vi "DHT.vi"() -> ()   [LabVIEW 2024]
uses:
  <vilib>/MakerHub/LINX/Public/Utilities/Open Serial.vi
  <vilib>/MakerHub/LINX/LMH-LINX.lvlib
panel:
  in  "FOLDER REPORTS":path
  in  "SAVE DATA":bool
  out "TOTAL ALARM OF HUM":dbl
  out "TOTAL ALARM OF TEMP":dbl
  out "REAL TIME TEMPERATURE C°":u8
  out "REAL TIME HUMIDITY %":u8
  out "ALLARME UMIDITA'":bool
  out "ALLARME TEMPERATURA":bool
  in  "INF HUMIDITY %":u16
  in  "SUP HUMIDITY %":u16
  in  "INF TEMPERATURE C°":u16
  in  "SUP TEMPERATURE C°":u16
  out "SAMPLES ACQUISITI":u16
  out "MODA T C°":dbl
  out "MINIMO T C°":dbl
  out "MODA H%":dbl
  out "MINIMO H%":dbl
  in  "SAMPLE TIME [ms]":u16=100 min=100
  out "MASSIMO T C°":dbl
  out "DEV STD T":dbl
  out "MEDIA T C°":dbl
  out "MASSIMO H%":dbl
  out "DEV STD H":dbl
  out "MEDIA H%":dbl
  out "HUMIDITY %":u8[](graph)
  out "TEMPERATURE C°":u8[](graph)
  out "COMUNICATION":string
  out "TEMPERATURE C°":u8(graph)
  out "HUMIDITY %":u8(graph)
  in  "NUMERO DI CAMPIONI":u16
  in  "ACQUIRE":bool
  in  "stop":bool
  in  "Serial Port":refnum<visa-resource-name>="N/A"
  # "SOGLIE"
  # "PARAMETRI STATISTICI TEMPERATURA"
  # "PARAMETRI STATISTICI UMIDITA'"
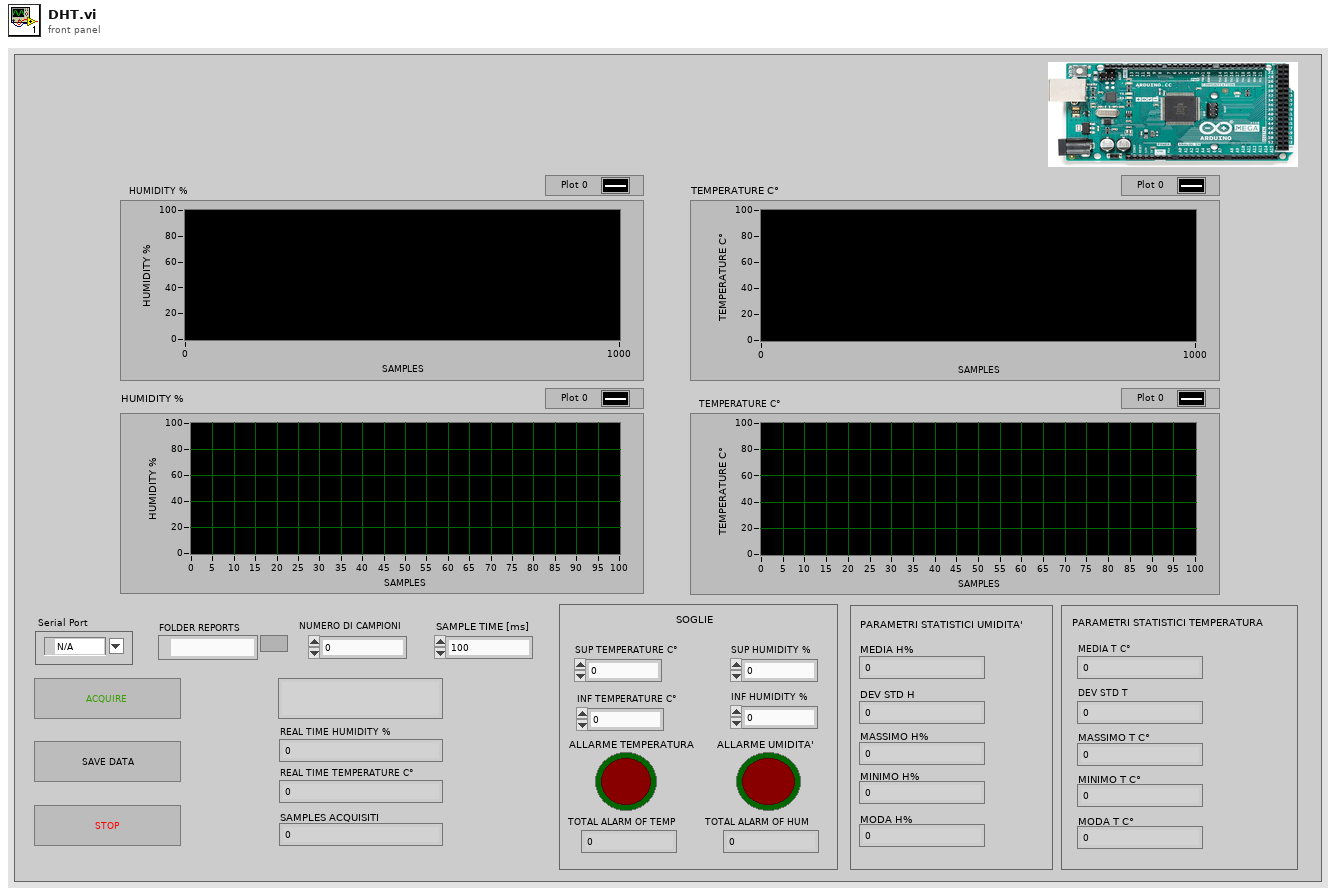
[diagram p1: front panel]
types:
  T1 = typedef "LMH-LINX.lvlib/LINX Ref.ctl" = cluster{"IO":T2, "Interface":T3, "LINX Device Config":T4}
  T2 = typedef "LMH-LINX.lvlib/Platform.ctl" = enum16{"Remote", "Local"}
  T3 = typedef "LMH-LINX.lvlib/Interface.ctl" = enum16{"Serial", "TCP"}
  T4 = typedef "LMH-LINX.lvlib/Device.lvlib/LINX Device Config.ctl" = cluster{"Interface":T3, "COM Port":refnum<visa-resource-name>, "TCP Configuration":T5, "Device Family":u8, "Device ID":u8, "Device Name":string, "TCP Ref":refnum<k5>, "Channels":T6}
  T5 = typedef "LMH-LINX.lvlib/Device.lvlib/TCP Config.ctl" = cluster{"IP Address":string, "Port":u16}
  T6 = typedef "LMH-LINX.lvlib/Channels.ctl" = cluster{"DI":u8[], "DO":u8[], "AI":u8[], "AO":u8[], "PWM":u8[], "QE":u8[], "UART":u8[], "I2C 2":u8[], "SPI":u8[], "CAN":u8[], "Servo":u8[], "AI Ref (V)":dbl, "AI Resolution (Bits)":u8, "AO Ref (V)":dbl, "AO Resolution (Bits)":u8}
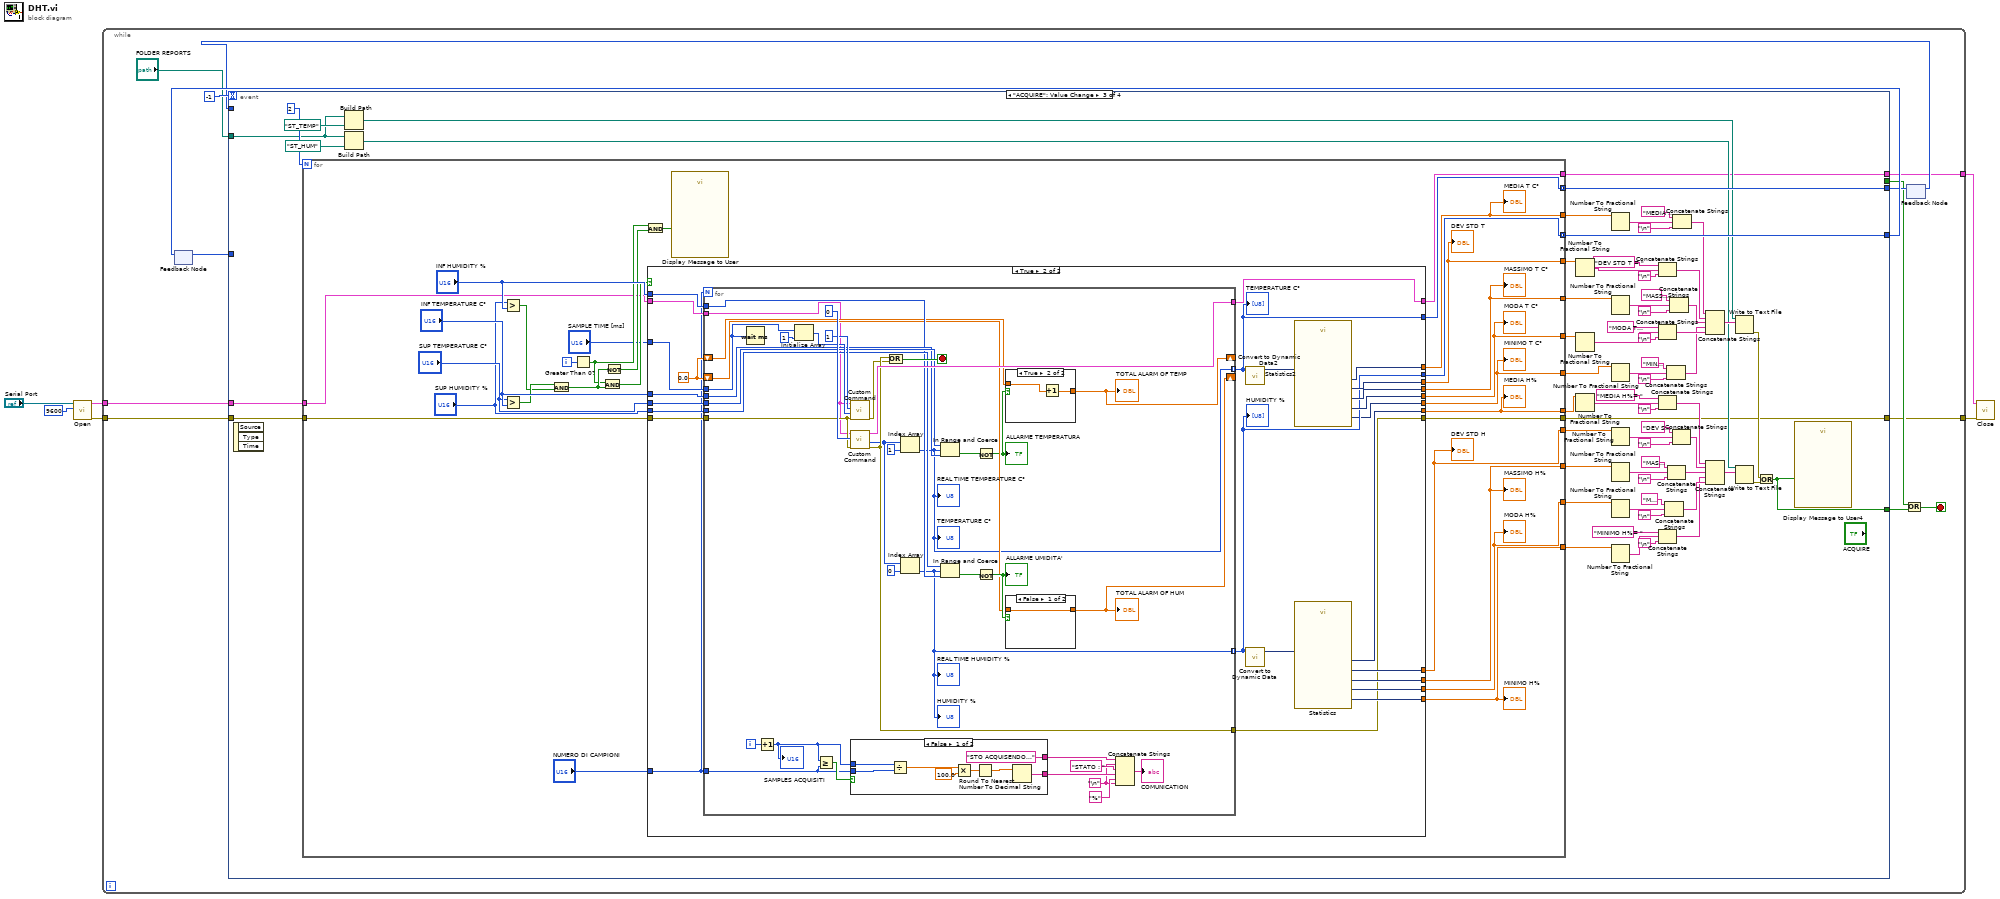
[diagram p0: block diagram]
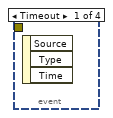
[diagram p2: hidden frame]
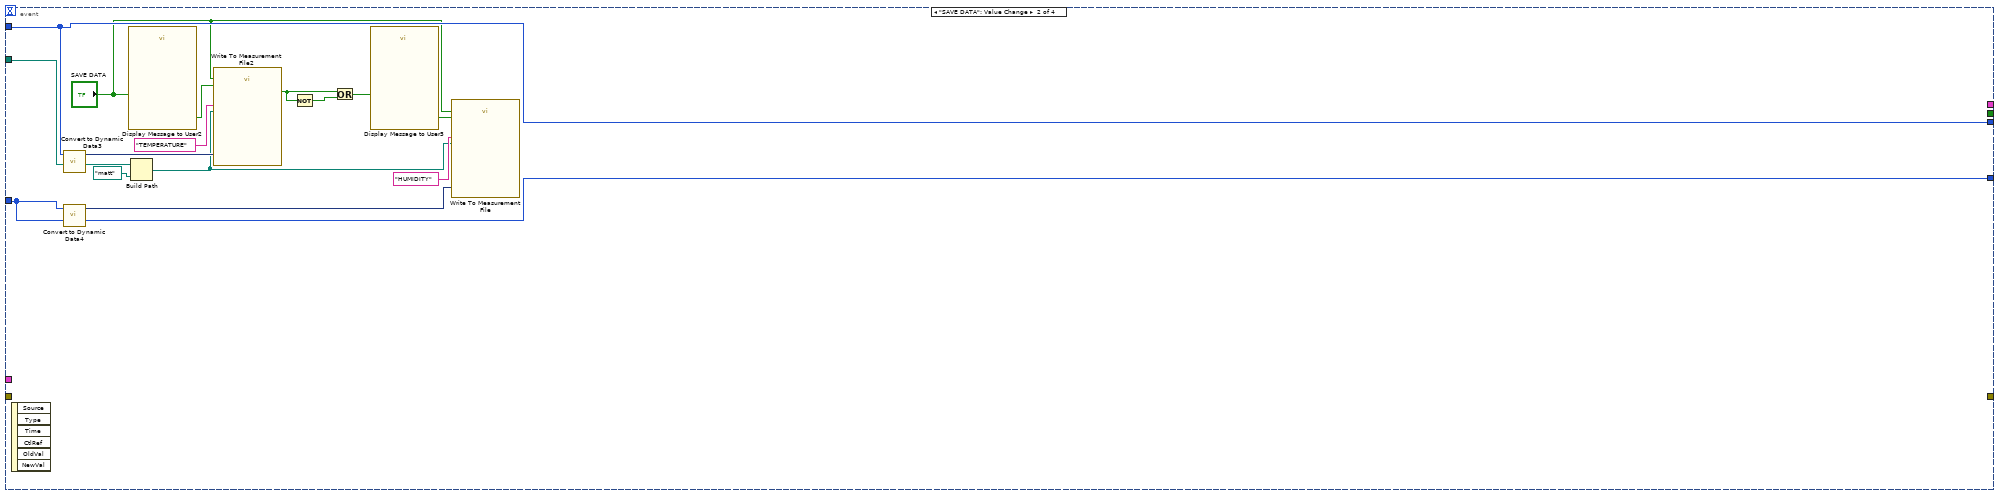
[diagram p3: hidden frame]
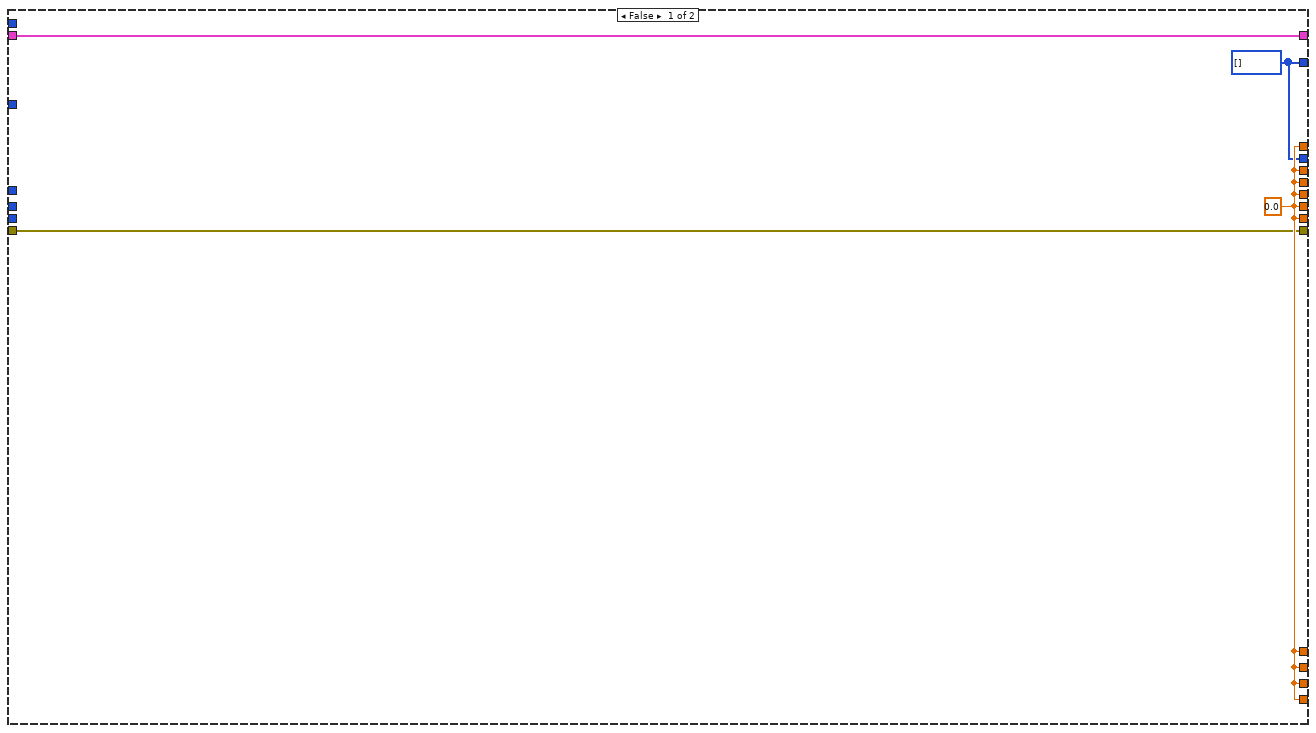
[diagram p4: hidden frame]
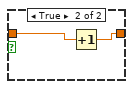
[diagram p6: hidden frame]
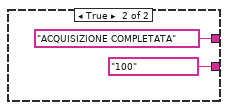
[diagram p7: hidden frame]
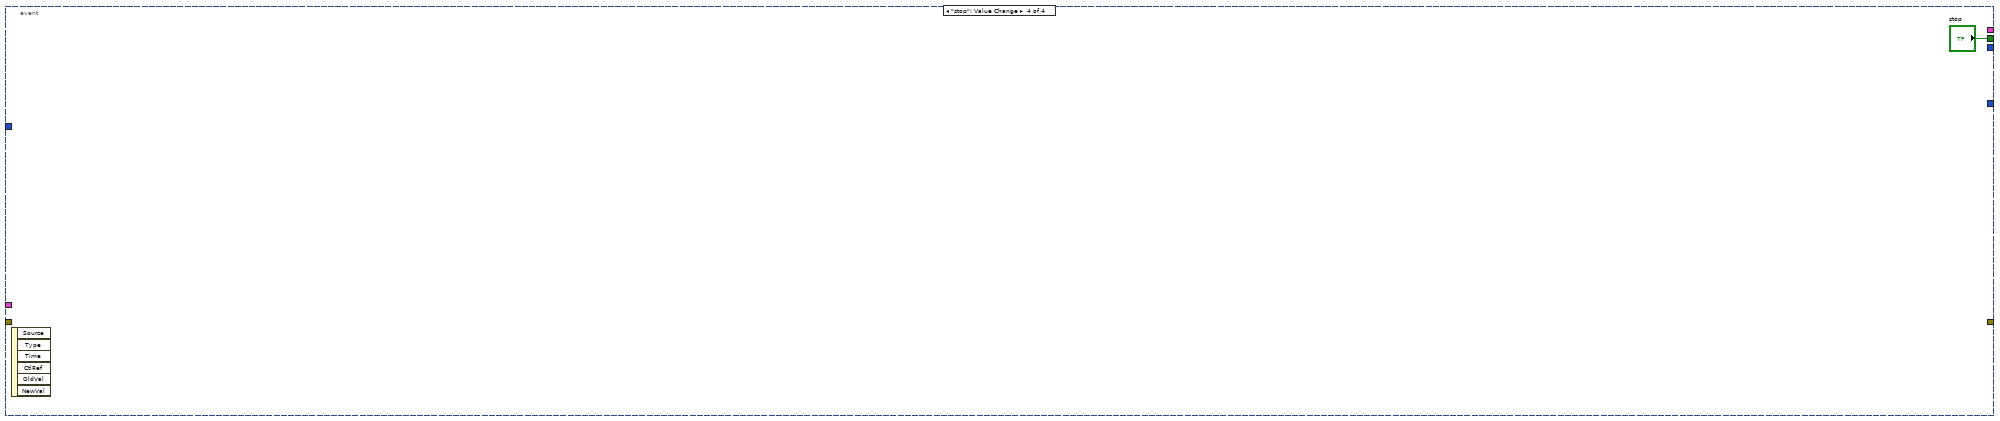
[diagram p8: hidden frame]
diagram:
  n1 = call-poly <vilib>:"Open.vi"("Baud Rate Override"=u32 9600, "Serial Port"="Serial Port") -> ("Error Out"=w2:errorcluster, "LINX Resource"=w1:T1)  [unwired: 7 in, 1 out]
  n2 = while {
    tunnel: [w10] -> w6
    tunnel: [w9] -> w5
    tunnel: w2 -> [w8]
    tunnel: w1 -> [w7]
    stop <- w12 stop-if-true
    n3 = feedback #1() -> (w17:u8[])  [unwired: 1 in]
    n4 = feedback #2() -> (w15:u8[])  [unwired: 1 in]
    n5 = event shown="[2] \"ACQUIRE\": Value Change" {
      selector: _ -> [_ _ _ _]
      dyn-events: _ -> [_ _ _ _]
      timeout: -1 -> [_ _ _ _]
      tunnel: [_ _ _ "stop"] -> w14
      tunnel: [_ w24 w100 _] -> w18
      tunnel: [_ w25 w99 _] -> w16
      tunnel: w17 -> [_ w24 _ _]
      tunnel: w15 -> [_ w25 _ _]
      tunnel: [_ _ w40 _] -> w13
      tunnel: "FOLDER REPORTS" -> [_ w23 w39 _]
      tunnel: w8 -> [_ _ w38 _]
      tunnel: w7 -> [_ _ w37 _]
      tunnel: [_ _ w36 _] -> w10
      tunnel: [_ _ w35 _] -> w9
      event Timeout {
        n6 = event-data() -> ()  [unwired: 1 in, 3 out]
      }
      event "SAVE DATA": Value Change {
        n7 = event-data() -> ()  [unwired: 1 in, 6 out]
        n8 = call "Convert to Dynamic Data3"("Array"=w25) -> ("Dynamic Data Type"=w27:dynamicdata)  [unwired: 3 in]
        n9 = call "Convert to Dynamic Data4"("Array"=w24) -> ("Dynamic Data Type"=w26:dynamicdata)  [unwired: 3 in]
        n10 = call "Display Message to User2"("Enable"="SAVE DATA") -> ("OK"=w32:bool)  [unwired: 9 in, 1 out]
        n11 = Build Path(base path=w23, name or relative path=path "matt") -> (appended path=w21:path)
        n12 = call "Write To Measurement File2"("Signals"=w27, "Reset"="SAVE DATA", "Enable"=w32, "Filename"=w21, "Comment"="TEMPERATURE") -> ("Saving Data"=w28:bool)  [unwired: 12 in, 2 out]
        n13 = Not(x=w28) -> (.not. x?=w29:bool)
        n14 = Or(x=w28, y=w29) -> (x .or. y?=w30:bool)
        n15 = call "Display Message to User3"("Enable"=w30) -> ("OK"=w31:bool)  [unwired: 9 in, 1 out]
        n16 = call "Write To Measurement File"("Signals"=w26, "Reset"="SAVE DATA", "Enable"=w31, "Filename"=w21, "Comment"="HUMIDITY") -> ()  [unwired: 12 in, 3 out]
      }
      event "ACQUIRE": Value Change {
        n17 = event-data() -> ()  [unwired: 1 in, 3 out]
        n18 = for {
          N: 2 -> [_]
          tunnel: [w130] -> w100 mode=concatenating
          tunnel: [w129] -> w99 mode=concatenating
          tunnel: [w128] -> w57
          tunnel: [w127] -> w60
          tunnel: [w126] -> w63
          tunnel: [w125] -> w66
          tunnel: [w124] -> w69
          tunnel: [w123] -> w72
          tunnel: [w122] -> w75
          tunnel: [w121] -> w78
          tunnel: [w120] -> w81
          tunnel: [w119] -> w84
          tunnel: w38 -> [w107]
          tunnel: w37 -> [w106]
          tunnel: [w103] -> w36
          tunnel: [w102] -> w35
          i -> [w131]
          n19 = Greater?(x="SUP HUMIDITY %", y="INF HUMIDITY %") -> (0:w113:bool)
          n20 = Greater?(x="SUP TEMPERATURE C°", y="INF TEMPERATURE C°") -> (0:w114:bool)
          n21 = And(x=w114, y=w113) -> (x .and. y?=w112:bool)
          n22 = Greater Than 0?(x=w131) -> (x > 0?=w110:bool)
          n23 = And(x=w110, y=w112) -> (x .and. y?=w111:bool)
          n24 = Not(x=w112) -> (.not. x?=w109:bool)
          n25 = And(x=w110, y=w109) -> (x .and. y?=w108:bool)
          n26 = case shown="True" w111 {
            tunnel: [w135 w158] -> w128
            tunnel: [w135 w152] -> w126
            tunnel: [w135 w146] -> w125
            tunnel: [w135 w157] -> w119
            tunnel: [w135 w147] -> w120
            tunnel: [w135 w156] -> w121
            tunnel: [w135 w155] -> w123
            tunnel: [w135 w154] -> w122
            tunnel: [w135 w153] -> w127
            tunnel: [w135 w151] -> w124
            tunnel: [w134 w149] -> w130
            tunnel: [w134 w148] -> w129
            tunnel: "INF TEMPERATURE C°" -> [_ w144]
            tunnel: "SUP TEMPERATURE C°" -> [_ w145]
            tunnel: "INF HUMIDITY %" -> [_ w142]
            tunnel: "SUP HUMIDITY %" -> [_ w143]
            tunnel: w107 -> [w132 w141]
            tunnel: w106 -> [w133 w140]
            tunnel: "SAMPLE TIME [ms]" -> [_ w139]
            tunnel: "NUMERO DI CAMPIONI" -> [_ w138]
            tunnel: [w132 w137] -> w103
            tunnel: [w133 w136] -> w102
            frame False {
              w134 = u8[] []
              w135 = 0.0
            }
            frame True {
              w150 = 0.0
              n27 = for {
                N: w138 -> [_]
                tunnel: [w198] -> w136
                tunnel: [w196] -> w137
                tunnel: w138 -> [w189]
                tunnel: [w167] -> w149 mode=indexing
                tunnel: [w164] -> w148 mode=indexing
                tunnel: w139 -> [w163]
                tunnel: w145 -> [w180]
                tunnel: w144 -> [w179]
                tunnel: w143 -> [w178]
                tunnel: w142 -> [w177]
                shift-right: [w169] -> _
                shift-left: w150 -> [w171]
                shift-right: [w170] -> _
                shift-left: w150 -> [w173]
                tunnel: w141 -> [w162]
                tunnel: w140 -> [w161]
                i -> [w192]
                stop <- w186 stop-if-true
                w181 = "\n"
                n28 = Wait (ms)(milliseconds to wait=w163) -> ()  [unwired: 1 out]
                n29 = Increment(x=w192) -> (x+1=w185:i32)
                "SAMPLES ACQUISITI" <- w185
                n30 = Initialize Array(w163, 1 ("dimension size")) -> (w190:u16[])
                n31 = Greater Or Equal?(x=w185, y=w189) -> (x >= y?=w193:bool)
                n32 = call <vilib>:"Custom Command.vi"("Error In"=w162, "Data"=w190, "Custom Command Number"=u16 1, "LINX Resource"=w161) -> ("Error Out"=w194:errorcluster)  [unwired: 4 in, 3 out]
                n33 = call <vilib>:"Custom Command.vi"("Error In"=w162, "Custom Command Number"=u16 0, "LINX Resource"=w161) -> ("Error Out"=w196:errorcluster, "Response"=w165:u8[], "LINX Resource"=w198:T1)  [unwired: 5 in, 1 out]
                n34 = case shown="False" w193 {
                  tunnel: ["STO ACQUISENDO..." ("COMUNICATION") "ACQUISIZIONE COMPLETATA" ("COMUNICATION")] -> w188
                  tunnel: w189 -> [w210 _]
                  tunnel: w185 -> [w211 _]
                  tunnel: [w205 "100" ("type")] -> w183
                  frame False {
                    n35 = Divide(x=w211, y=w210) -> (x/y=w209:dbl)
                    n36 = Multiply(x=w209, y=100.0) -> (x*y=w207:dbl)
                    n37 = Round To Nearest(number=w207) -> (nearest integer value=w206:dbl)
                    n38 = Number To Decimal String(number=w206) -> (decimal integer string=w205:string)  [unwired: 1 in]
                  }
                  frame True {
                  }
                }
                n39 = Or(x=w196, y=w194) -> (x .or. y?=w186:bool)
                n40 = Index Array(array=w165, index=1) -> (element=w164:u8)
                "TEMPERATURE C°" <- w164
                "REAL TIME TEMPERATURE C°" <- w164
                n41 = Index Array(array=w165, index=0) -> (element=w167:u8)
                "HUMIDITY %" <- w167
                "REAL TIME HUMIDITY %" <- w167
                n42 = In Range and Coerce(upper limit=w180, x=w164, lower limit=w179) -> (In Range?=w176:bool)  [unwired: 1 out]
                n43 = In Range and Coerce(upper limit=w178, x=w167, lower limit=w177) -> (In Range?=w175:bool)  [unwired: 1 out]
                n44 = Not(x=w176) -> (.not. x?=w172:bool)
                "ALLARME TEMPERATURA" <- w172
                n45 = Not(x=w175) -> (.not. x?=w174:bool)
                "ALLARME UMIDITA'" <- w174
                n46 = case shown="True" w172 {
                  tunnel: w171 -> [w199 w201]
                  tunnel: [w199 w200] -> w169
                  frame False {
                  }
                  frame True {
                    n47 = Increment(x=w201) -> (x+1=w200:dbl)
                  }
                }
                "TOTAL ALARM OF TEMP" <- w169
                n48 = case shown="False" w174 {
                  tunnel: w173 -> [w202 w204]
                  tunnel: [w202 w203] -> w170
                  frame False {
                  }
                  frame True {
                    n49 = Increment(x=w204) -> (x+1=w203:dbl)
                  }
                }
                "TOTAL ALARM OF HUM" <- w170
                n50 = Concatenate Strings(w188, w181, "STATO : " ("string"), w183, "%" ("string"), w181) -> (→"COMUNICATION":string)
              }
              "TEMPERATURE C°" <- w148
              "HUMIDITY %" <- w149
              n51 = call "Convert to Dynamic Data2"("Array"=w148) -> ("Dynamic Data Type"=w159:dynamicdata)  [unwired: 3 in]
              n52 = call "Convert to Dynamic Data"("Array"=w149) -> ("Dynamic Data Type"=w160:dynamicdata)  [unwired: 3 in]
              n53 = call "Statistics2"("Signals"=w159) -> ("Mode"=w157:dynamicdata, "Standard Dev"=w154:dynamicdata, "Arithmetic Mean"=w155:dynamicdata, "Minimum"=w147:dynamicdata, "Maximum"=w156:dynamicdata)  [unwired: 21 in, 1 out]
              n54 = call "Statistics"("Signals"=w160) -> ("Mode"=w151:dynamicdata, "Standard Dev"=w153:dynamicdata, "Arithmetic Mean"=w158:dynamicdata, "Minimum"=w146:dynamicdata, "Maximum"=w152:dynamicdata)  [unwired: 21 in, 1 out]
            }
          }
          "MEDIA H%" <- w128
          "DEV STD H" <- w127
          "MASSIMO H%" <- w126
          "MINIMO H%" <- w125
          "MODA H%" <- w124
          "DEV STD T" <- w122
          "MEDIA T C°" <- w123
          "MASSIMO T C°" <- w121
          "MINIMO T C°" <- w120
          "MODA T C°" <- w119
          n55 = call "Display Message to User"("Enable"=w108) -> ()  [unwired: 9 in, 2 out]
        }
        n56 = Build Path(base path=w39, name or relative path=path "ST_TEMP") -> (appended path=w45:path)
        n57 = Build Path(base path=w39, name or relative path=path "ST_HUM") -> (appended path=w43:path)
        n58 = Number To Fractional String(number=w75) -> (F-format string=w50:string)  [unwired: 3 in]
        n59 = Number To Fractional String(number=w84) -> (F-format string=w47:string)  [unwired: 3 in]
        n60 = Number To Fractional String(number=w57) -> (F-format string=w56:string)  [unwired: 3 in]
        n61 = Number To Fractional String(number=w72) -> (F-format string=w51:string)  [unwired: 3 in]
        n62 = Number To Fractional String(number=w78) -> (F-format string=w49:string)  [unwired: 3 in]
        n63 = Number To Fractional String(number=w81) -> (F-format string=w48:string)  [unwired: 3 in]
        n64 = Number To Fractional String(number=w60) -> (F-format string=w55:string)  [unwired: 3 in]
        n65 = Number To Fractional String(number=w63) -> (F-format string=w54:string)  [unwired: 3 in]
        n66 = Number To Fractional String(number=w69) -> (F-format string=w52:string)  [unwired: 3 in]
        n67 = Number To Fractional String(number=w66) -> (F-format string=w53:string)  [unwired: 3 in]
        n68 = Concatenate Strings("DEV STD T = " ("string"), w50, "\n") -> (w88:string)
        n69 = Concatenate Strings("MODA T C°= " ("string"), w47, "\n") -> (w91:string)
        n70 = Concatenate Strings("MEDIA H%= " ("string"), w56, "\n") -> (w92:string)
        n71 = Concatenate Strings("MINIMO H%= " ("string"), w53, "\n") -> (w95:string)
        n72 = Concatenate Strings("MODA H%= " ("string"), w52, "\n") -> (w96:string)
        n73 = Concatenate Strings("MINIMO T C°= " ("string"), w48, "\n") -> (w90:string)
        n74 = Concatenate Strings("MASSIMO H%= " ("string"), w54, "\n") -> (w94:string)
        n75 = Concatenate Strings("MASSIMO T C°= " ("string"), w49, "\n") -> (w89:string)
        n76 = Concatenate Strings("DEV STD H= " ("string"), w55, "\n") -> (w93:string)
        n77 = Concatenate Strings("MEDIA T C°= " ("string"), w51, "\n") -> (w87:string)
        n78 = Concatenate Strings(w87, w88, w89, w90, w91) -> (w98:string)
        n79 = Concatenate Strings(w92, w93, w94, w95, w96) -> (w97:string)
        n80 = Write to Text File(file (use dialog)=w45, text=w98) -> (error out=w42:errorcluster)  [unwired: 2 in, 2 out]
        n81 = Write to Text File(file (use dialog)=w43, text=w97) -> (error out=w41:errorcluster)  [unwired: 2 in, 2 out]
        n82 = Or(x=w42, y=w41) -> (x .or. y?=w40:bool)
        n83 = call "Display Message to User4"("Enable"=w40) -> ()  [unwired: 9 in, 2 out]
      }
      event "stop": Value Change {
        n84 = event-data() -> ()  [unwired: 1 in, 6 out]
      }
    }
    n85 = feedback-in #1(w18) -> ()
    n86 = Or(x=w14, y=w13) -> (x .or. y?=w12:bool)
    n87 = feedback-in #2(w16) -> ()
  }
  n88 = call <vilib>:"Close.vi"("Error In"=w6, "LINX Resource"=w5) -> ()  [unwired: 9 in, 1 out]
